vi "OpenNIVeriStand.vi"(8 "error in (no error)":errorcluster) -> (0 "error out":errorcluster)   [LabVIEW 2015]
uses:
  NationalInstruments.VeriStand.Internal
  <vilib>/NI Veristand/Execution/Workspace/NI_VS Workspace ExecutionAPI.lvlib
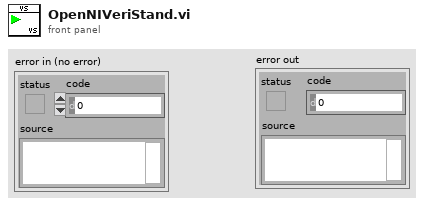
[diagram p1: front panel]
types:
  T1 = typedef "NI_VS Workspace ExecutionAPI.lvlib/WorkspaceAPI.ctl" = refnum<k24>
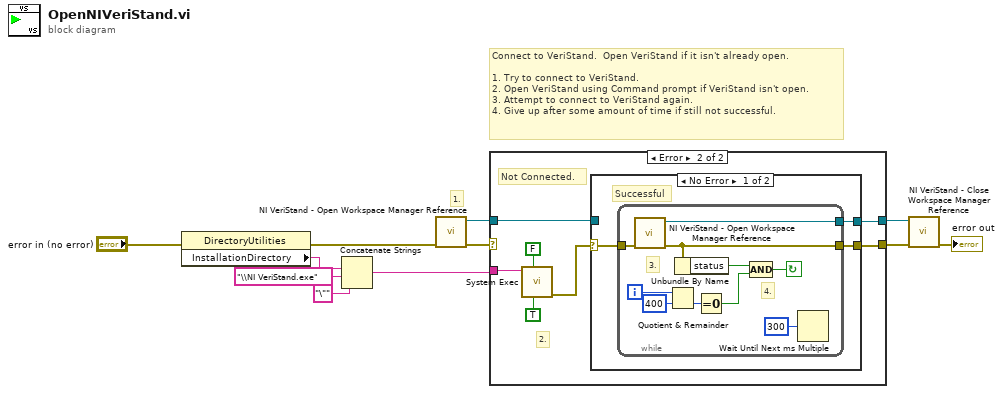
[diagram p0: block diagram]
diagram:
  w1 = "\"" ("string")
  # "1."
  # "Connect to VeriStand.  Open VeriStand if it isn't already open.\n\n1. Try to connect to VeriStand.\n2. Open VeriStand using Command prompt if VeriStand isn't open.\n3. Attempt to connect to VeriStand again.\n4. Give up after some amount of time if still not successful."
  n1 = property class="DirectoryUtilities"(error in="error in (no error)") -> (error out=w2:errorcluster, "InstallationDirectory"=w9:string)  [unwired: 1 in, 1 out]
  n2 = Concatenate Strings(w1, w9, "\\NI VeriStand.exe" ("string"), w1) -> (w4:string)
  n3 = call <vilib>:"NI VeriStand - Open Workspace Manager Reference.vi"("error in (no error)"=w2) -> ("error out"=w10:errorcluster, "WorkspaceManager"=w11:T1)  [unwired: 9 in]
  n4 = case shown="Error" w10 {
    selector: w10 -> [w12 _]
    tunnel: w11 -> [w13 w18]
    tunnel: [w13 w17] -> w6
    tunnel: [w12 w16] -> w7
    tunnel: w4 -> [_ w14]
    frame No Error {
      # "Connected"
    }
    frame Error {
      # "2."
      # "Not Connected."
      n5 = call <vilib>:"System Exec.vi"("run minimized? (F)"=TRUE, "wait until completion? (T)"=FALSE, "command line"=w14) -> ("error out"=w19:errorcluster)  [unwired: 5 in, 3 out]
      n6 = case shown="No Error" w19 {
        selector: w19 -> [w21 w34]
        tunnel: [w23 w35] -> w17
        tunnel: [w22 w34] -> w16
        tunnel: w18 -> [_ w35]
        frame No Error {
          # "Successful"
          n7 = while {
            tunnel: [w33] -> w23
            tunnel: [w31] -> w22
            tunnel: w21 -> [w30]
            i -> [w28]
            stop <- w26 continue-if-true
            # "4."
            # "3."
            n8 = call <vilib>:"NI VeriStand - Open Workspace Manager Reference.vi"("error in (no error)"=w30) -> ("error out"=w31:errorcluster, "WorkspaceManager"=w33:T1)  [unwired: 9 in]
            n9 = Quotient & Remainder(x=w28, y=400) -> (floor(x/y)=w25:i32)  [unwired: 1 out]
            n10 = Unbundle By Name(w31) -> ("status"=w29:bool)
            n11 = Equal To 0?(x=w25) -> (x = 0?=w24:bool)
            n12 = Compound Arithmetic op=AND(w29, w24) -> (w26:bool)
            n13 = Wait Until Next ms Multiple(millisecond multiple=u32 300) -> ()  [unwired: 1 out]
          }
        }
        frame Error {
          # "Not Successful.  Pass Error."
        }
      }
    }
  }
  n14 = call <vilib>:"NI VeriStand - Close Workspace Manager Reference.vi"("error in (no error)"=w7, "WorkspaceManager"=w6) -> ("error out"=→"error out":errorcluster)  [unwired: 9 in]
